vi "Close_queue_and_com.vi"(11 "VISA":refnum<visa-resource-name>) -> ()   [LabVIEW 2017]
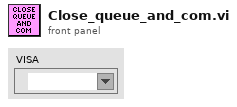
[diagram p1: front panel]
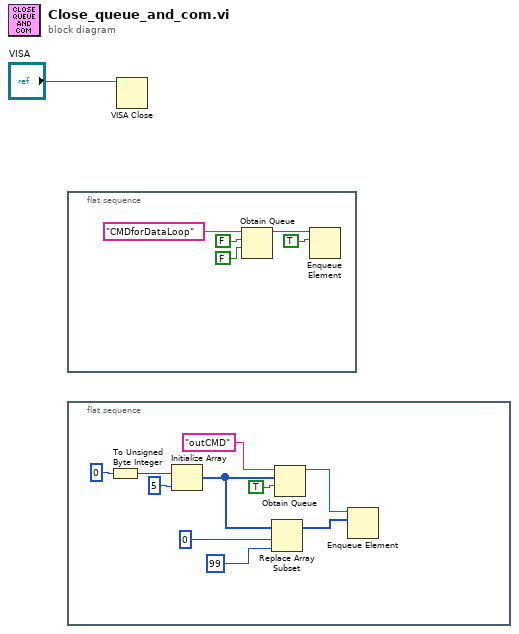
[diagram p0: block diagram]
diagram:
  n1 = flat-sequence {
    frame #0 {
      n2 = Obtain Queue(name (unnamed)="CMDforDataLoop", element data type=FALSE ("create if not found? (T)"), create if not found? (T)=FALSE) -> (queue out=w3:refnum<queue>)  [unwired: 2 in, 2 out]
      n3 = Enqueue Element(queue=w3, element=TRUE) -> ()  [unwired: 2 in, 3 out]
    }
  }
  n4 = flat-sequence {
    frame #0 {
      n5 = To Unsigned Byte Integer(number=u8 0) -> (unsigned 8bit integer=w15:u8)
      n6 = Initialize Array(w15, 5 ("dimension size")) -> (w11:u8[])
      n7 = Replace Array Subset(array=w11, new element=u8 99 ("new element/subarray"), index=0) -> (w7:u8[])
      n8 = Obtain Queue(name (unnamed)="outCMD", element data type=w11, create if not found? (T)=TRUE) -> (queue out=w8:refnum<queue>)  [unwired: 2 in, 2 out]
      n9 = Enqueue Element(queue=w8, element=w7) -> ()  [unwired: 2 in, 3 out]
    }
  }
  n10 = VISA Close(VISA resource name="VISA") -> ()  [unwired: 1 in, 1 out]
